vi "test-CSM mode.vi"(8 "error in (no error)":errorcluster, 11 "TestCase in":refnum<class "testcase-CSMAttributes.lvclass">) -> (0 "error out":errorcluster, 3 "TestCase out":refnum<class "testcase-CSMAttributes.lvclass">)   [LabVIEW 2017, in "testcase-CSMAttributes.lvclass"]
uses:
  testcase-CSMAttributes.lvclass
  5e1fa0b9-9953-4aea-b14f-852d0926f464.vi
  ca6da20f-918c-4697-94f5-fe779df5fb56.vi
  b6cafa74-5be5-493d-85c2-392da22f0834.vi
  474ebc5b-ede4-4fe2-a33b-3b2c34e901f1.vi
  6dc37769-ead1-45fc-a673-d21298543349.vi
  2b38d03e-680a-4e35-9447-0bd23ed7c194.vi
  aa53e100-d513-4525-b5da-2cac676b671d.vi
  src/user.lib/_NEVSTOP/Communicable State Machine(CSM)/AdvanceAPI/CSM - Set Module Attribute.vi
  src/user.lib/_NEVSTOP/Communicable State Machine(CSM)/AdvanceAPI/CSM - Get Module Attribute.vi
  <vilib>/addons/_JKI Toolkits/VI Tester/TestCase.llb/TestCase.lvclass
  src/user.lib/_NEVSTOP/Communicable State Machine(CSM)/Communicable State Machine.lvlib
  C:/Program Files (x86)/National Instruments/LabVIEW 2017/vi.lib/addons/_JKI Toolkits/VI Tester/TestCase.llb/TestCase.lvclass
panel:
  out "error out":errorcluster
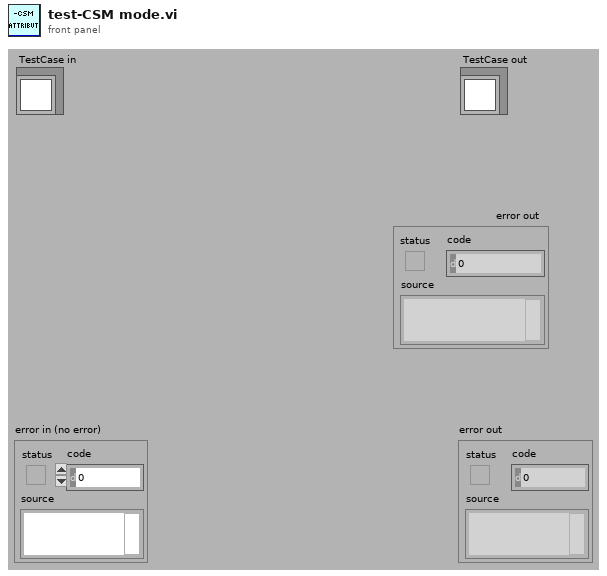
[diagram p1: front panel]
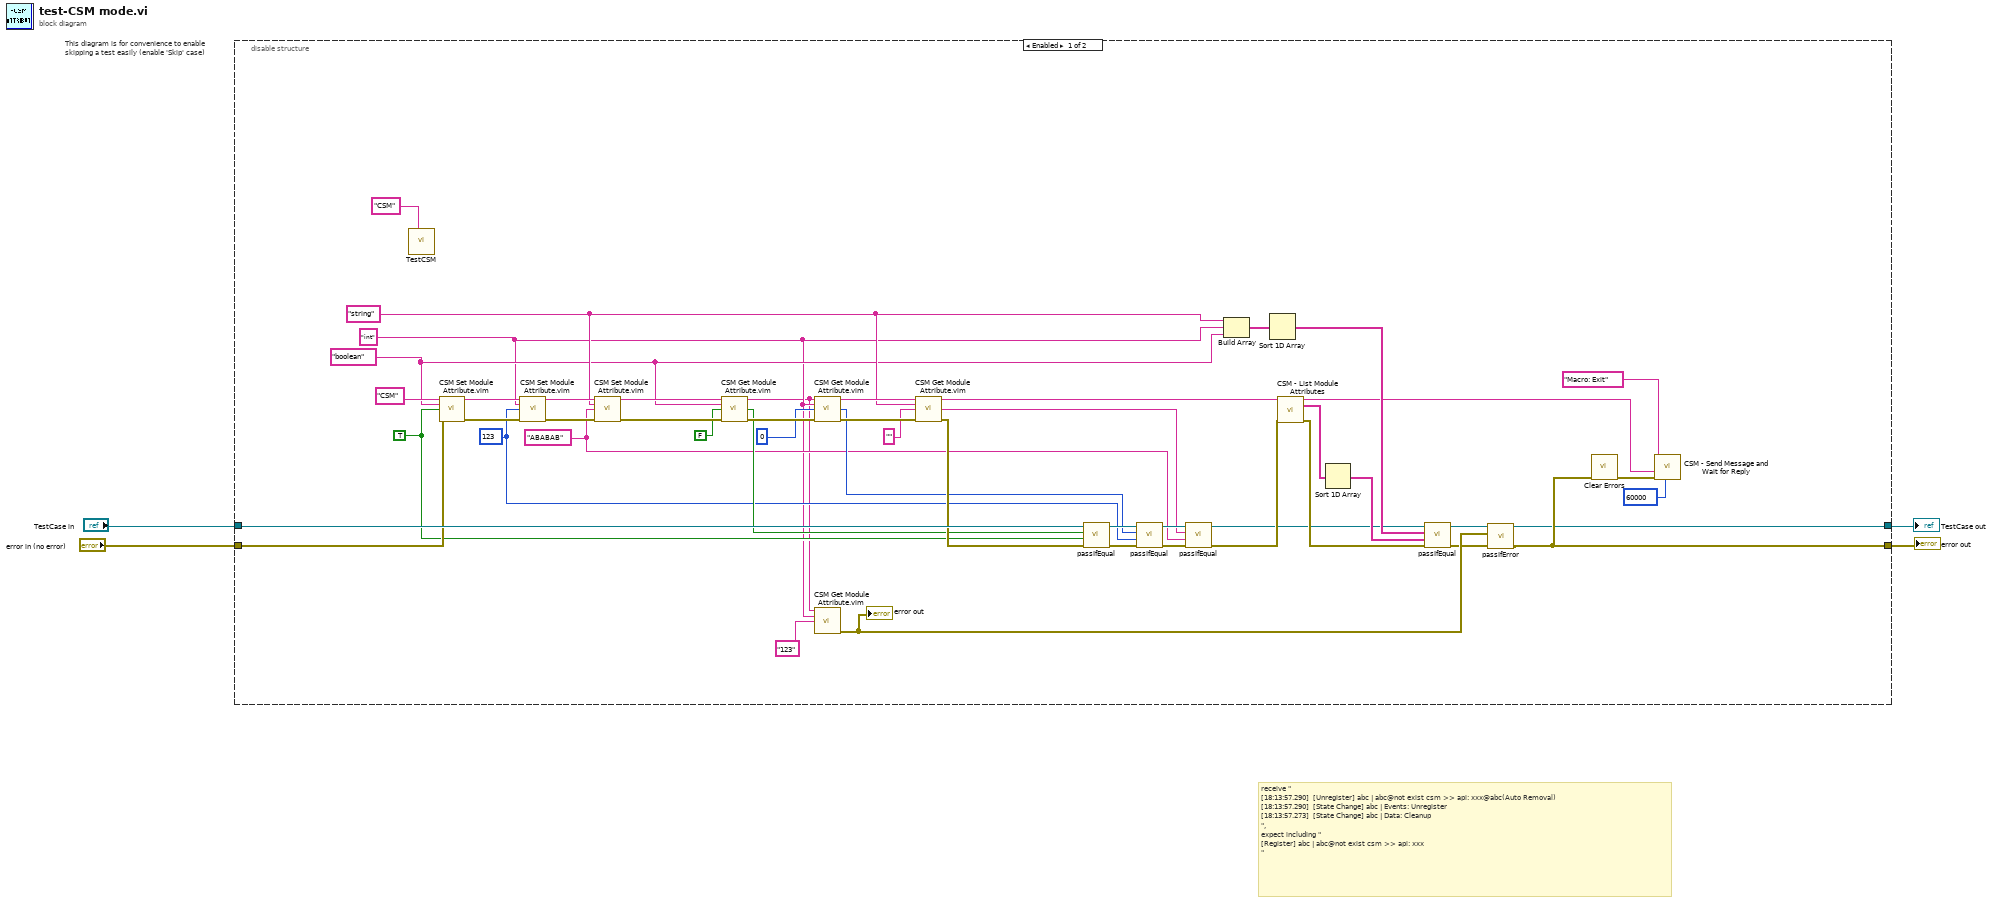
[diagram p0: block diagram]
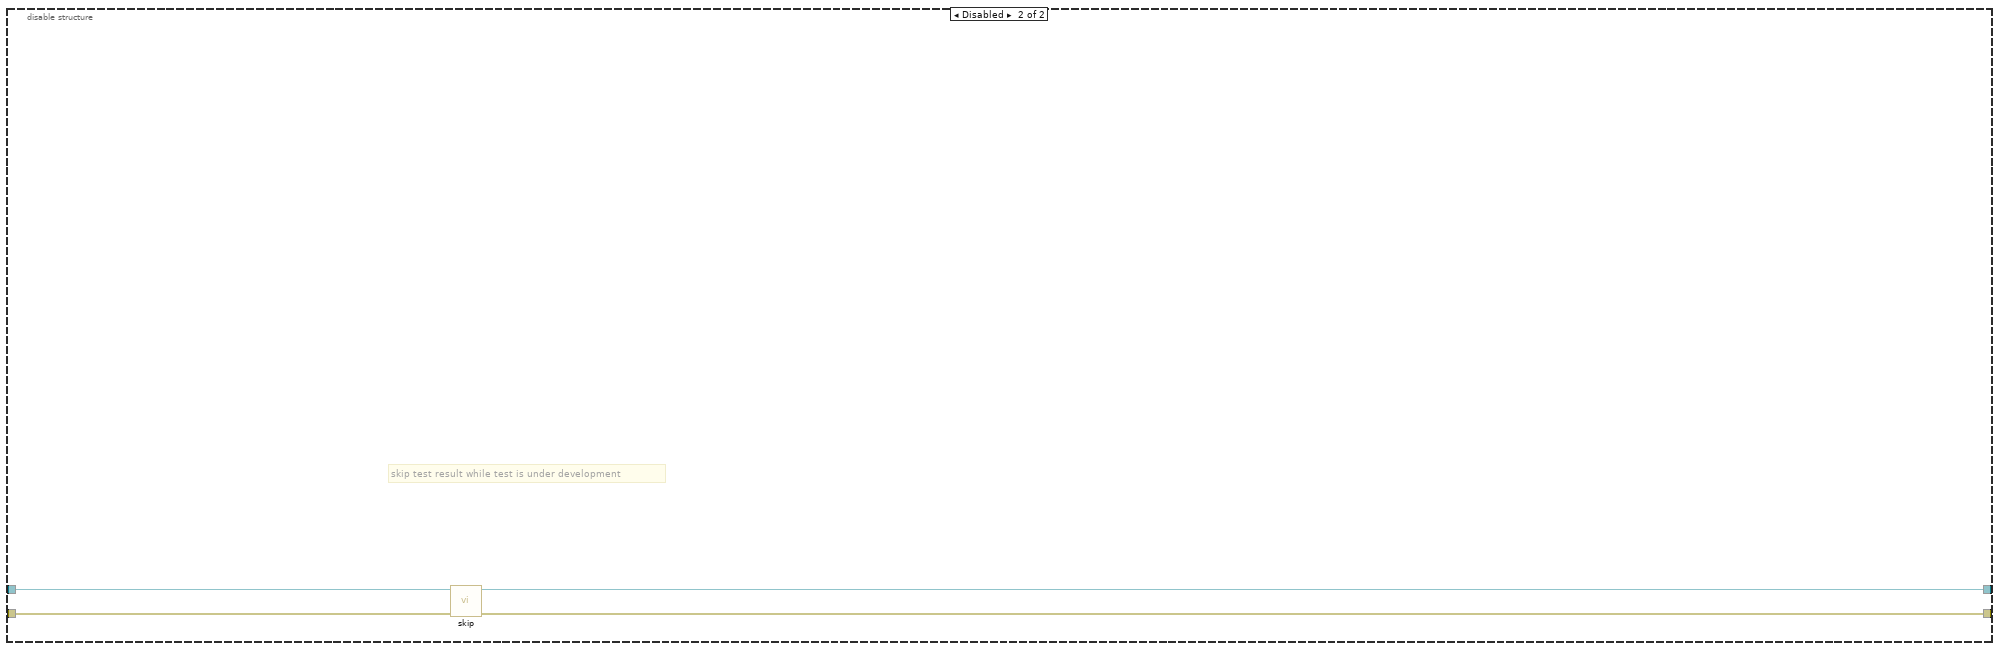
[diagram p2: hidden frame]
diagram:
  # "receive \"\n[18:13:57.290]  [Unregister] abc | abc@not exist csm >> api: xxx@abc(Auto Removal)\n[18:13:57.290]  [State Change] abc | Events: Unregister\n[18:13:57.273]  [State Change] abc | Data: Cleanup\n\", \nexpect including \"\n[Register] abc | abc@not exist csm >> api: xxx\n\""
  n1 = disable-structure "This diagram is for convenience to enable skipping a test easily (enable 'Skip' case)" shown="Enabled" {
    disable-tunnel: "TestCase in" -> [w53 w57]
    disable-tunnel: [w6 w55] -> w1
    disable-tunnel: [w7 w56] -> w3
    disable-tunnel: "error in (no error)" -> [w52 w54]
    frame Enabled {
      w27 = "ABABAB" ("Attribute")
      w23 = "string" ("Attribute")
      w31 = 123
      w12 = "int" ("Attribute")
      w36 = TRUE
      w22 = "boolean" ("Attribute")
      n2 = call "TestCSM.vi"("Name (\"\" to Use UUID)"="CSM" ("Name (\"\" to Use UUID)")) -> ()  [unwired: 11 in]
      n3 = call "CSM Set Module Attribute.vim"("CSM Name"="CSM" ("Name (\"\" to Use UUID)"), "Attribute"=w22, "Value"=w36, "Error In"=w52) -> ("CSM Name (Dup)"=w47:string, "error out"=w49:errorcluster)  [unwired: 8 in, 2 out]
      n4 = call "CSM Set Module Attribute.vim"("CSM Name"=w47, "Attribute"=w12, "Value"=w31, "Error In"=w49) -> ("CSM Name (Dup)"=w46:string, "error out"=w48:errorcluster)  [unwired: 8 in, 2 out]
      n5 = call "CSM Set Module Attribute.vim"("CSM Name"=w46, "Attribute"=w23, "Value"=w27, "Error In"=w48) -> ("CSM Name (Dup)"=w44:string, "error out"=w45:errorcluster)  [unwired: 8 in, 2 out]
      n6 = call "CSM Get Module Attribute.vim"("CSM Name"=w44, "Attribute"=w22, "Default Value (Empty Variant)"=FALSE, "Error In"=w45) -> ("CSM Name (Dup)"=w11:string, "Value"=w35:bool, "error out"=w43:errorcluster)  [unwired: 7 in, 2 out]
      n7 = call "CSM Get Module Attribute.vim"("CSM Name"=w11, "Attribute"=w12, "Default Value (Empty Variant)"=0, "Error In"=w43) -> ("CSM Name (Dup)"=w42:string, "Value"=w32:i32, "error out"=w41:errorcluster)  [unwired: 7 in, 2 out]
      n8 = call "CSM Get Module Attribute.vim"("CSM Name"=w11, "Attribute"=w12, "Default Value (Empty Variant)"="123") -> ("error out"=w9:errorcluster)  [unwired: 8 in, 4 out]
      "error out" <- w9
      n9 = call "CSM Get Module Attribute.vim"("CSM Name"=w42, "Attribute"=w23, "Default Value (Empty Variant)"="" ("Attribute"), "Error In"=w41) -> ("CSM Name (Dup)"=w26:string, "Value"=w28:string, "error out"=w37:errorcluster)  [unwired: 7 in, 2 out]
      n10 = call-dynamic "passIfEqual.vi"("error in (no error)"=w37, "y"=w36, "x"=w35, "TestCase in"=w53) -> ("error out"=w33:errorcluster, "TestCase out"=w34:refnum<class "testcase-CSMAttributes.lvclass">)  [unwired: 6 in]
      n11 = call-dynamic "passIfEqual.vi"("error in (no error)"=w33, "y"=w31, "x"=w32, "TestCase in"=w34) -> ("error out"=w29:errorcluster, "TestCase out"=w30:refnum<class "testcase-CSMAttributes.lvclass">)  [unwired: 6 in]
      n12 = call-dynamic "passIfEqual.vi"("error in (no error)"=w29, "y"=w27, "x"=w28, "TestCase in"=w30) -> ("error out"=w25:errorcluster, "TestCase out"=w17:refnum<class "testcase-CSMAttributes.lvclass">)  [unwired: 6 in]
      n13 = Build Array(w23, w12, w22) -> (w21:string[])
      n14 = Sort 1D Array(array=w21) -> (sorted array=w18:string[])
      n15 = call "CSM - List Module Attributes.vi"("CSM Name"=w26, "Error In"=w25) -> ("CSM Name (Dup)"=w15:string, "Attributes"=w20:string[], "error out"=w24:errorcluster)  [unwired: 9 in, 2 out]
      n16 = Sort 1D Array(array=w20) -> (sorted array=w19:string[])
      n17 = call-dynamic "passIfEqual.vi"("error in (no error)"=w24, "y"=w19, "x"=w18, "TestCase in"=w17) -> ("error out"=w8:errorcluster, "TestCase out"=w10:refnum<class "testcase-CSMAttributes.lvclass">)  [unwired: 6 in]
      n18 = call-dynamic "passIfError.vi"("error in (no error)"=w8, "error"=w9, "TestCase in"=w10) -> ("error out"=w7:errorcluster, "TestCase out"=w6:refnum<class "testcase-CSMAttributes.lvclass">)  [unwired: 7 in]
      n19 = call <vilib>:"Clear Errors.vi"("error in (no error)"=w7) -> ("error out"=w16:errorcluster)  [unwired: 5 in, 1 out]
      n20 = call "CSM - Send Message and Wait for Reply.vi"("Response Timeout (-2 Using Global Settings)"=60000, "Error In (No Error)"=w16, "Target Module"=w15, "State"="Macro: Exit") -> ()  [unwired: 5 in, 3 out]
    }
    frame Disabled {
      # "skip test result while test is under development"
      n21 = call <vilib>:"skip.vi"("error in (no error)"=w54, "TestCase in"=w57) -> ("error out"=w56:errorcluster, "TestCase out"=w55:refnum<class "testcase-CSMAttributes.lvclass">)  [unwired: 8 in]
    }
  }
  "error out" <- w3
  "TestCase out" <- w1
